vi "Update all channels.vi"(8 "Error In":errorcluster, 9 "Value":sgl min=0 max=204.8 step=0.0125 format="%#_g V", 11 "Arduino Port":refnum<visa-resource-name>) -> (0 "Error Out":errorcluster, 3 "Arduino Port out":refnum<visa-resource-name>)   [LabVIEW 2016]
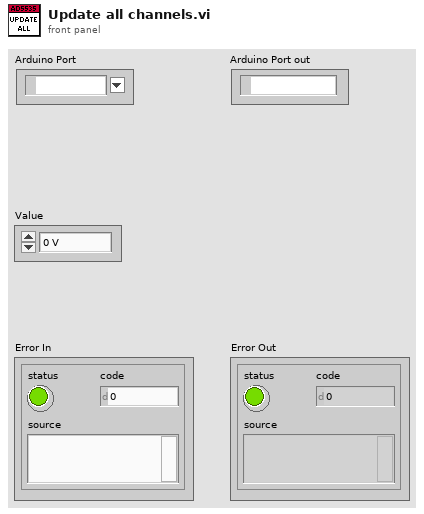
[diagram p1: front panel]
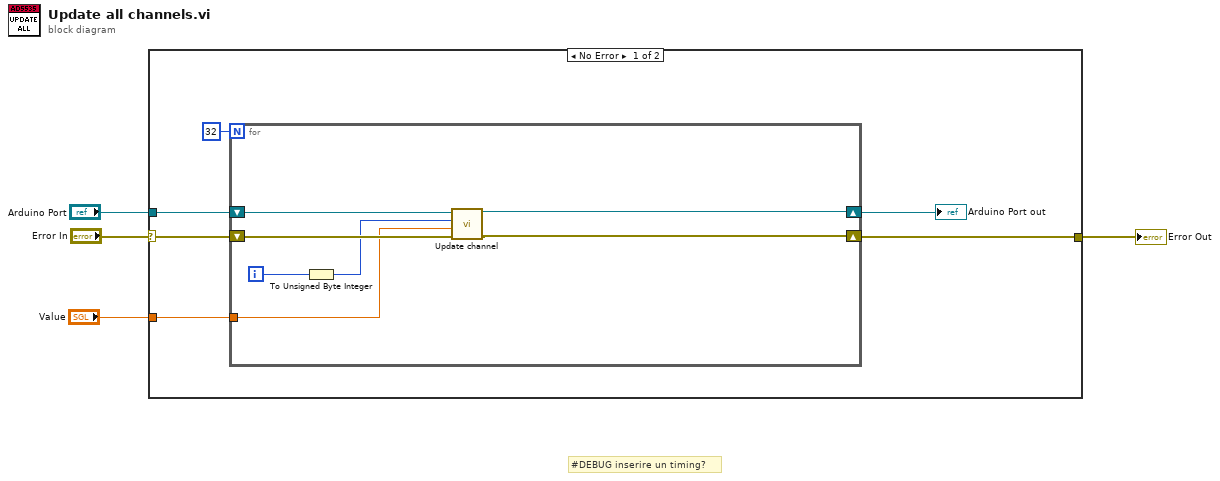
[diagram p0: block diagram]
diagram:
  # "#DEBUG inserire un timing?"
  n1 = case shown="No Error" "Error In" {
    selector: "Error In" -> [w9 w18]
    tunnel: [w8 w18] -> w3
    tunnel: "Arduino Port" -> [w10 _]
    tunnel: "Value" -> [w6 _]
    frame No Error {
      n2 = for {
        N: 32 -> [_]
        tunnel: w6 -> [w13]
        shift-right: [w12] -> w7
        shift-left: w10 -> [w16]
        shift-right: [w11] -> w8
        shift-left: w9 -> [w15]
        i -> [w17]
        n3 = To Unsigned Byte Integer(number=w17) -> (unsigned 8bit integer=w14:u8)
        n4 = call "Update channel.vi"("Error In"=w15, "Value"=w13, "Channel"=w14, "Arduino Port"=w16) -> ("Error Out"=w11:errorcluster, "Arduino Port out"=w12:refnum<visa-resource-name>)  [unwired: 6 in]
      }
      "Arduino Port out" <- w7
    }
    frame Error {
    }
  }
  "Error Out" <- w3
